vi "Make from Project.vi"(8 "error in (no error)":errorcluster, 10 "Project Path":path, 11 "LUnit Test Suite In":refnum<class "LUnit Test Suite.lvclass">) -> (0 "error out":errorcluster, 3 "LUnit Test Suite Out":refnum<class "LUnit Test Suite.lvclass">)   [LabVIEW 2020, in "LUnit Test Suite.lvclass"]
uses:
  LUnit Test Suite.lvclass
  C:/Git/astemes-lunit/source/Core/Runnable/Runnable.lvclass
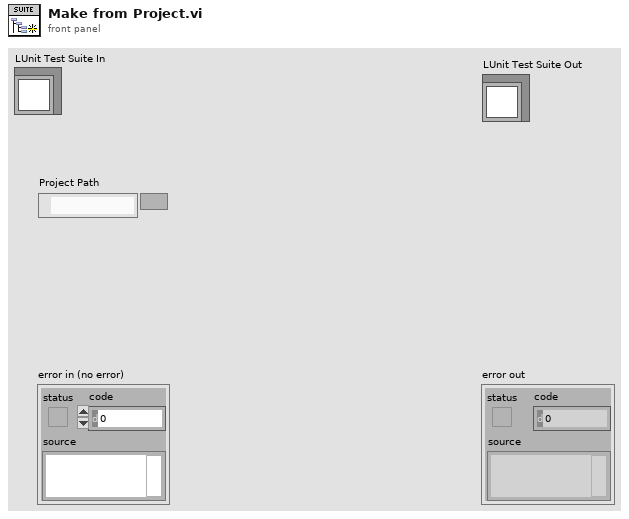
[diagram p1: front panel]
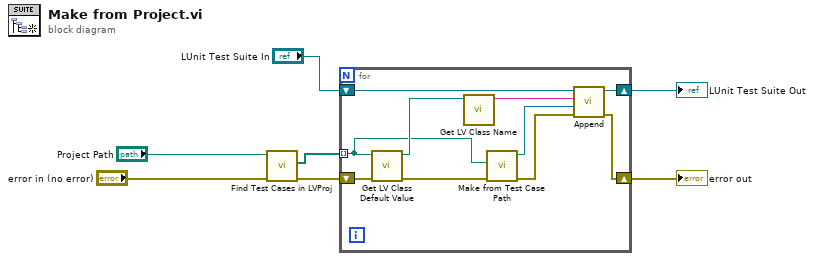
[diagram p0: block diagram]
diagram:
  n1 = call "Find Test Cases in LVProj.vi"("error in (no error)"="error in (no error)", "Project Path"="Project Path") -> ("error out"=w5:errorcluster, "Test Class paths"=w6:path[])  [unwired: 8 in]
  n2 = for {
    tunnel: w6 -> [w11] mode=indexing
    shift-right: [w15] -> w1
    shift-left: "LUnit Test Suite In" -> [w16]
    shift-right: [w14] -> w3
    shift-left: w5 -> [w17]
    n3 = call <vilib>:"Get LV Class Default Value.vi"("error in (no error)"=w17, "class path"=w11) -> ("error out"=w10:errorcluster, "object"=w13:refnum<class>)  [unwired: 8 in]
    n4 = call <vilib>:"Get LV Class Name.vi"("object"=w13) -> ("class name"=w12:string)  [unwired: 9 in, 1 out]
    n5 = call "Make from Test Case Path.vi"("error in (no error)"=w10, "Test Case"=w11) -> ("error out"=w9:errorcluster, "LUnit Test Suite Out"=w8:refnum<class "LUnit Test Suite.lvclass">)  [unwired: 8 in]
    n6 = call "Append.vi"("error in (no error)"=w9, "Runnable"=w8, "Name"=w12, "LUnit Test Suite In"=w16) -> ("error out"=w14:errorcluster, "LUnit Test Suite Out"=w15:refnum<class "LUnit Test Suite.lvclass">)  [unwired: 6 in]
  }
  "error out" <- w3
  "LUnit Test Suite Out" <- w1
